vi "StartStop.vi"(8 "error in (no error)":errorcluster, 10 "Start/Stop":bool, 11 "Counter in":refnum<class "Counter.lvclass">) -> (0 "error out":errorcluster, 3 "Counter out":refnum<class "Counter.lvclass">)   [LabVIEW 2019, in "Counter.lvlib" / "Counter.lvclass"]
uses:
  Counter.lvclass
  Counter.lvclass/Counter.ctl
  Counter ACQ Messages/StartStop Msg/StartStop Msg.lvclass/StartStop Msg.ctl
  <vilib>/ActorFramework/Message Enqueuer/Message Enqueuer.lvclass/Message Enqueuer.ctl
  <vilib>/ActorFramework/Message Enqueuer/Enqueue.vi
  Counter ACQ Messages/StartStop Msg/StartStop Msg.lvclass
  C:/Program Files/National Instruments/LabVIEW 2019/vi.lib/ActorFramework/Message/Message.lvclass
  <vilib>/ActorFramework/Message Priority Queue/Priority Enqueue.vi
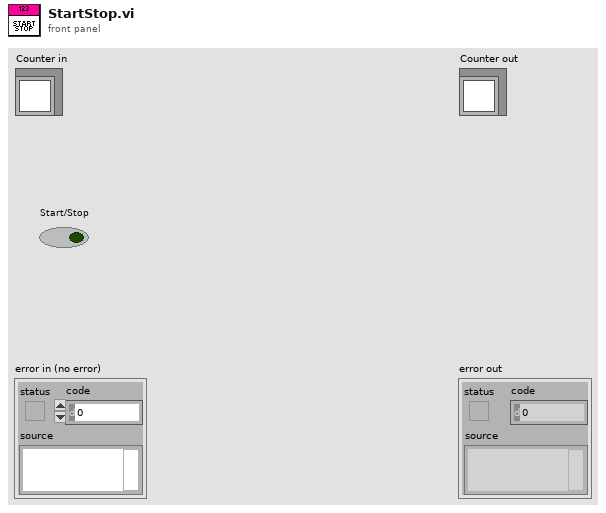
[diagram p1: front panel]
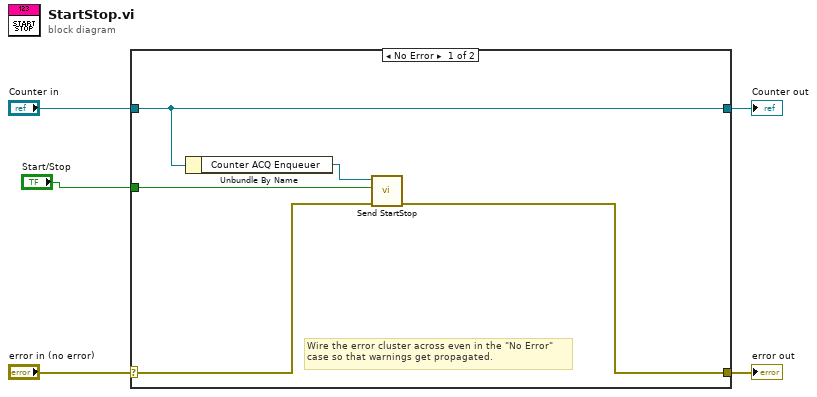
[diagram p0: block diagram]
diagram:
  n1 = case shown="No Error" "error in (no error)" {
    selector: "error in (no error)" -> [w7 w12]
    tunnel: [w6 w12] -> w4
    tunnel: [w9 w11] -> w2
    tunnel: "Counter in" -> [w9 w11]
    tunnel: "Start/Stop" -> [w10 _]
    frame No Error {
      # "Wire the error cluster across even in the \"No Error\"\ncase so that warnings get propagated."
      n2 = Unbundle By Name(w9) -> ("Counter ACQ Enqueuer"=w8:refnum<class "Message Enqueuer.lvclass">)
      n3 = call "Send StartStop.vi"("error in (no error)"=w7, "Start/Stop"=w10, "Message Enqueuer"=w8) -> ("error out"=w6:errorcluster)  [unwired: 7 in, 1 out]
    }
    frame Error {
    }
  }
  "error out" <- w4
  "Counter out" <- w2
